vi "ConfigUtilities - Initialize Packet Page Panel.vi"(7 "Channels Listbox":refnum<vi>, 8 "error in (no error)":errorcluster, 9 "Channel Paths Property":string, 10 "Channel Names Property":string, 11 "Item Ref in":T1 format="%.0x") -> (0 "error out":errorcluster, 1 "Channel Paths":string[](array[string]), 2 "Channel Names":string[](array[string]), 3 "Item Ref out":T1 format="%.0x")   [LabVIEW 2016, in "UDP-Custom-Device System Explorer.lvlib"]
doc: "Initialize the Rx Channels Section Page Panel."
uses:
  UDP-Custom-Device System Explorer.lvlib
  <vilib>/NI Veristand/Custom Device API/Custom Device Item Ref.ctl
  <vilib>/Utility/miscctls.llb/LVRowAndColumnUnsignedTypeDef.ctl
  <vilib>/NI Veristand/Custom Device API/Get Item Property (String Array).vi
  <vilib>/NI VeriStand/Custom Device API/Custom Device API.lvlib
  Shared/UDP-Custom-Device Shared.lvlib
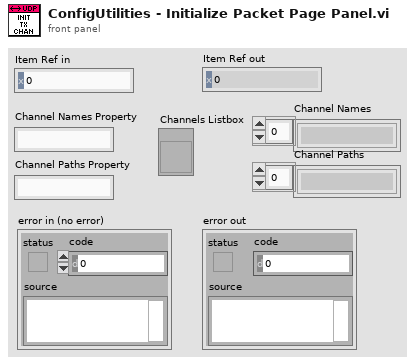
[diagram p1: front panel]
types:
  T1 = typedef "Custom Device API.lvlib/Custom Device Item Ref.ctl" = u64
  T2 = typedef "LVRowAndColumnUnsignedTypeDef.ctl" = cluster{"Row":u32, "Column":u32}
  T3 = typedef "UDP-Custom-Device Shared.lvlib/Channel Data Type.ctl" = enum16{"Boolean", "Single"}
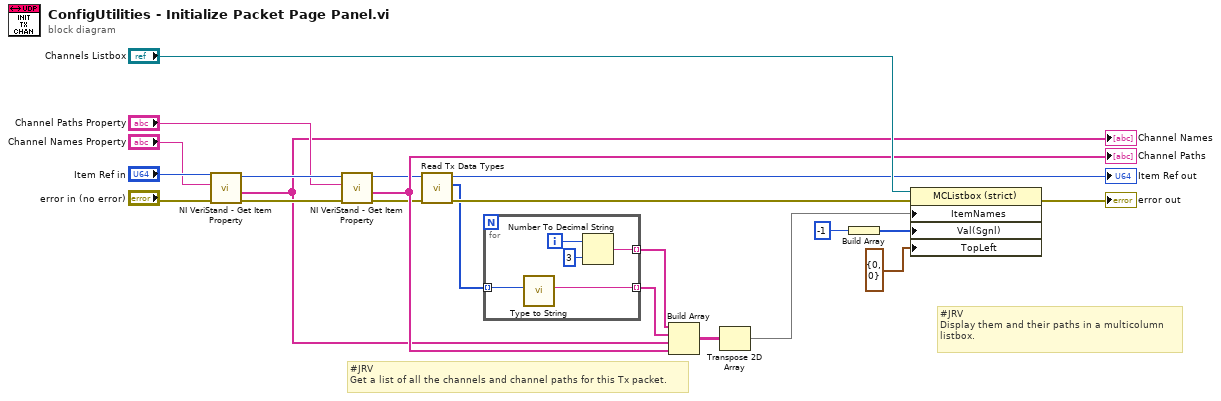
[diagram p0: block diagram]
diagram:
  # "#JRV\nDisplay them and their paths in a multicolumn\nlistbox."
  # "#JRV\nGet a list of all the channels and channel paths for this Tx packet."
  n1 = call-poly <vilib>:"NI VeriStand - Get Item Property.vi"("error in (no error)"="error in (no error)", "Property Name"="Channel Names Property", "Item Ref in"="Item Ref in") -> ("error out"=w17:errorcluster, "Value"=w8:string[], "Item Ref out"=w16:T1)  [unwired: 5 in, 1 out]
  "Channel Names" <- w8
  n2 = call-poly <vilib>:"NI VeriStand - Get Item Property.vi"("error in (no error)"=w17, "Property Name"="Channel Paths Property", "Item Ref in"=w16) -> ("error out"=w3:errorcluster, "Value"=w9:string[], "Item Ref out"=w5:T1)  [unwired: 5 in, 1 out]
  "Channel Paths" <- w9
  n3 = call "Read Tx Data Types.vi"("error in (no error)"=w3, "Node Ptr"=w5) -> ("error out"=w2:errorcluster, "Data types"=w1:T3[], "Node Ptr out"=→"Item Ref out":T1)  [unwired: 7 in]
  n4 = for {
    tunnel: [w23] -> w7 mode=indexing
    tunnel: [w25] -> w6 mode=indexing
    tunnel: w1 -> [w24] mode=indexing
    i -> [w27]
    n5 = call "Type to String.vi"("Data Type"=w24) -> ("String Type"=w23:string)  [unwired: 10 in]
    n6 = Number To Decimal String(number=w27, width (-)=i16 3) -> (decimal integer string=w25:string)
  }
  n7 = Build Array(w6, w7, w8, w9) -> (w18:string[][])
  n8 = Transpose 2D Array(2D array=w18) -> (transposed array=w20:string[][])
  n9 = Build Array(-1) -> (w21:i32[])
  n10 = property class="MCListbox (strict)"(reference="Channels Listbox", error in=w2, "ItemNames"=w20, "Val(Sgnl)"=w21, "TopLeft"=T2 {"Row"=0, "Column"=0} ("Top Left Visible Cell")) -> (error out=→"error out":errorcluster)  [unwired: 1 out]
